vi "8-bit video export-New file path-Auto increment.vi"(8 "error in (no error)":errorcluster, 11 "AVI modes refs":T1) -> (0 "error out":errorcluster, 3 "AVI modes refs":T1)   [LabVIEW 2020]
uses:
  Typedefs/8-bit video export AVI modes cluster.ctl
  <vilib>/vision/Avi1.llb/AviRefnum.ctl
  <vilib>/vision/Avi.llb/IMAQ AVI2 Refnum.ctl
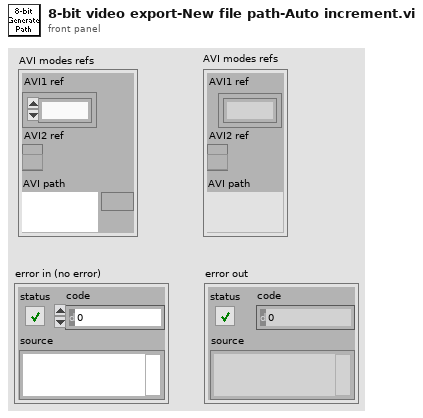
[diagram p1: front panel]
types:
  T1 = typedef "8-bit video export AVI modes cluster.ctl" = cluster{"AVI1 ref":T2, "AVI2 ref":T3, "AVI path":path}
  T2 = typedef "AviRefnum.ctl" = refnum<k1>
  T3 = typedef "IMAQ AVI2 Refnum.ctl" = refnum<k20>
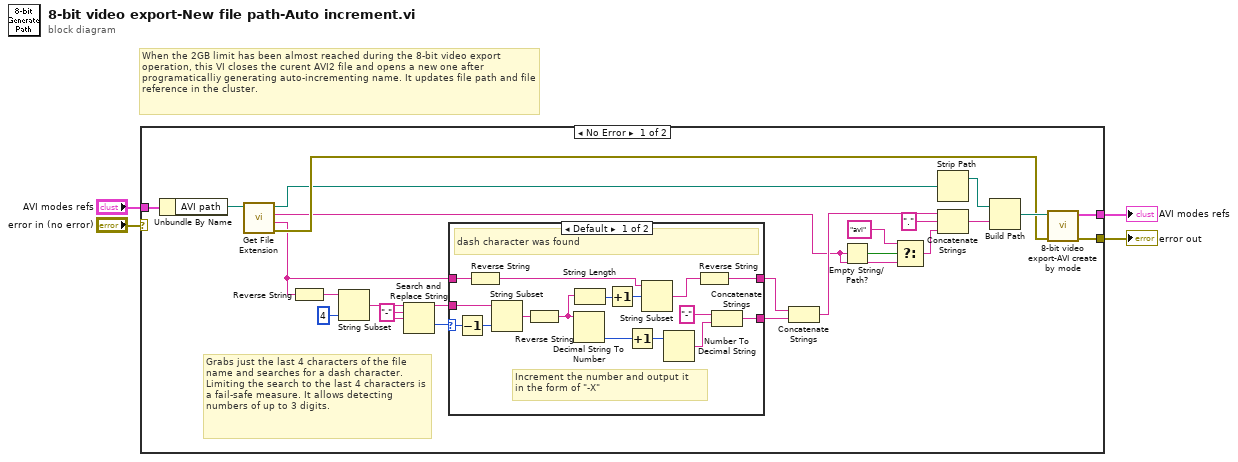
[diagram p0: block diagram]
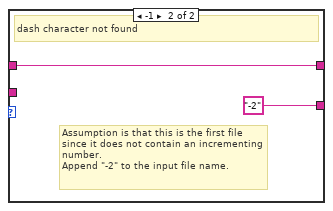
[diagram p2: hidden frame]
diagram:
  # "When the 2GB limit has been almost reached during the 8-bit video export operation, this VI closes the curent AVI2 file and opens a new one after programaticalliy generating auto-incrementing name. It updates file path and file reference in the cluster."
  n1 = case shown="No Error" "error in (no error)" {
    selector: "error in (no error)" -> [_ w48]
    tunnel: [w13 w48] -> w4
    tunnel: "AVI modes refs" -> [w27 w47]
    tunnel: [w28 w47] -> w1
    frame No Error {
      w25 = "-" ("search string")
      # "Grabs just the last 4 characters of the file name and searches for a dash character. Limiting the search to the last 4 characters is a fail-safe measure. It allows detecting numbers of up to 3 digits."
      n2 = Unbundle By Name(w27) -> ("AVI path"=w26:path)
      n3 = call <vilib>:"Get File Extension.vi"("file"=w26) -> ("error out"=w14:errorcluster, "filename without extension"=w8:string, "lowercase file extension"=w9:string, "dup file"=w6:path)  [unwired: 6 in, 1 out]
      n4 = Reverse String(1:w8) -> (0:w22:string)
      n5 = String Subset(string=w22, length (rest)=4 ("length (rest)")) -> (substring=w21:string)  [unwired: 1 in]
      n6 = Search and Replace String(input string=w21, search string=w25, replace string=w25) -> (result string=w23:string, offset past replacement=w24:i32)  [unwired: 5 in, 2 out]
      n7 = case shown="Default" w24 {
        selector: w24 -> [w43 _]
        tunnel: w23 -> [w44 _]
        tunnel: [w38 "-2" ("string")] -> w15
        tunnel: w8 -> [w33 w45]
        tunnel: [w30 w45] -> w7
        frame Default {
          # "Increment the number and output it\nin the form of \"-X\""
          # "dash character was found"
          n8 = Decrement(x=w43) -> (x-1=w36:i32)
          n9 = Reverse String(1:w33) -> (0:w32:string)
          n10 = String Subset(string=w44, length (rest)=w36) -> (substring=w42:string)  [unwired: 1 in]
          n11 = Reverse String(1:w42) -> (0:w35:string)
          n12 = Decimal String To Number(string=w35) -> (number=w41:i32)  [unwired: 2 in, 1 out]
          n13 = String Length(string=w35) -> (length=w34:i32)
          n14 = Increment(x=w34) -> (x+1=w29:i32)
          n15 = Increment(x=w41) -> (x+1=w40:i32)
          n16 = String Subset(string=w32, offset (0)=w29) -> (substring=w31:string)  [unwired: 1 in]
          n17 = Number To Decimal String(number=w40) -> (decimal integer string=w39:string)  [unwired: 1 in]
          n18 = Reverse String(1:w31) -> (0:w30:string)
          n19 = Concatenate Strings("-" ("string"), w39) -> (w38:string)
        }
        frame -1 {
          # "Assumption is that this is the first file since it does not contain an incrementing number.\nAppend \"-2\" to the input file name."
          # "dash character not found"
        }
      }
      n20 = Concatenate Strings(w7, w15) -> (w18:string)
      n21 = Empty String/Path?(string/path=w9) -> (empty?=w12:bool)
      n22 = Select(t="avi", s=w12, f=w9) -> (s? t:f=w11:string)
      n23 = Strip Path(path=w6) -> (stripped path=w5:path)  [unwired: 1 out]
      n24 = Concatenate Strings(w18, "." ("string"), w11) -> (w17:string)
      n25 = Build Path(base path=w5, name or relative path=w17) -> (appended path=w16:path)
      n26 = call "8-bit video export-AVI create by mode.vi"("error in (no error)"=w14, "8-bit AVI file path"=w16) -> ("error out"=w13:errorcluster, "AVI modes refs"=w28:T1)  [unwired: 8 in]
    }
    frame Error {
    }
  }
  "error out" <- w4
  "AVI modes refs" <- w1
